vi "Format Display to Uncertainty.vi"(5 "- uncertainty reference":refnum<vi>, 7 "+ uncertainty reference":refnum<vi>, 8 "error in (no error)":errorcluster, 11 "value reference":refnum<vi>) -> (0 "error out":errorcluster, 3 "formatting string":string)   [LabVIEW 2013, in "varilib.lvlib"]
doc: "Sets format of referenced numeric control according the positive or both positive or negative uncertainties of referenced numeric controls. Format is done to the order of two significant numbers of smaller uncertainty. A formatting string is returned in the output."
uses:
  varilib.lvlib
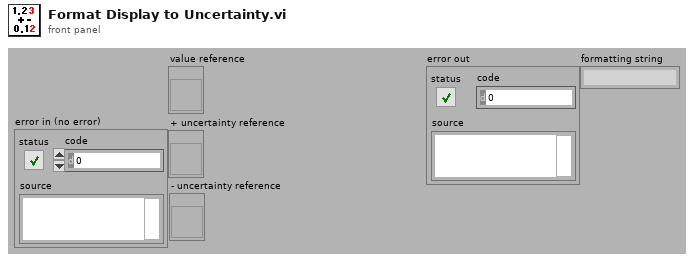
[diagram p1: front panel]
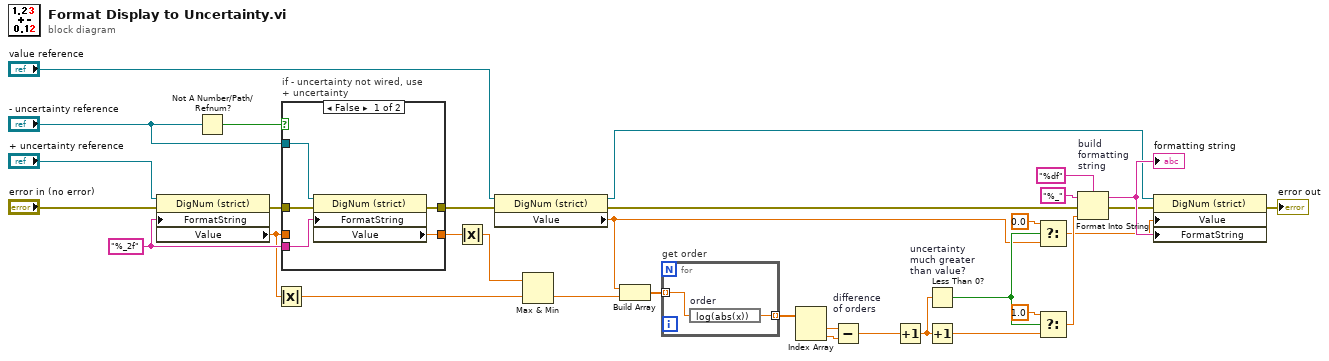
[diagram p0: block diagram]
diagram:
  w16 = "%_2f" ("Format String")
  n1 = property class="DigNum (strict)"(reference="+ uncertainty reference", error in="error in (no error)", "FormatString"=w16) -> (error out=w9:errorcluster, "Value"=w2:dbl)  [unwired: 1 out]
  n2 = Not A Number/Path/Refnum?(number/path/refnum="- uncertainty reference") -> (NaN/Path/Refnum?=w3:bool)
  n3 = Absolute Value(x=w2) -> (abs(x)=w14:dbl)
  n4 = case "if - uncertainty not wired, use \n+ uncertainty" shown="False" w3 {
    tunnel: w16 -> [w38 _]
    tunnel: [w37 w39] -> w15
    tunnel: w9 -> [w36 w40]
    tunnel: [w35 w40] -> w8
    tunnel: w2 -> [_ w39]
    tunnel: "- uncertainty reference" -> [w34 _]
    frame False {
      n5 = property class="DigNum (strict)"(reference=w34, error in=w36, "FormatString"=w38) -> (error out=w35:errorcluster, "Value"=w37:dbl)  [unwired: 1 out]
    }
    frame True {
    }
  }
  n6 = Absolute Value(x=w15) -> (abs(x)=w30:dbl)
  n7 = property class="DigNum (strict)"(reference="value reference", error in=w8) -> (reference out=w11:refnum<vi>, error out=w7:errorcluster, "Value"=w12:dbl)
  n8 = Max & Min(x=w30, y=w14) -> (min(x,y)=w13:dbl)  [unwired: 1 out]
  n9 = Build Array(w12, w13) -> (w27:dbl[])
  n10 = for "get order" {
    tunnel: [w41] -> w26 mode=indexing
    tunnel: w27 -> [w42] mode=indexing
    n11 = expression code="log(abs(x))" "order"(w42) -> (w41:dbl)
  }
  n12 = Index Array(array=w26) -> (element #1=w25:dbl, element #2=w24:dbl)  [unwired: 2 in]
  n13 = Subtract "difference\nof orders"(x=w25, y=w24) -> (x-y=w23:dbl)
  n14 = Increment(x=w23) -> (x+1=w17:dbl)
  n15 = Less Than 0? "uncertainty\nmuch greater\nthan value?"(x=w17) -> (x < 0?=w20:bool)
  n16 = Increment(x=w17) -> (x+1=w19:dbl)
  n17 = Select(t=0.0, s=w20, f=w12) -> (s? t:f=w10:dbl)
  n18 = Select(t=1.0, s=w20, f=w19) -> (s? t:f=w21:dbl)
  n19 = Format Into String "build\nformatting\nstring"(format string="%df", initial string="%_", error in=w7, w21) -> (resulting string=w31:string, error out=w6:errorcluster)
  "formatting string" <- w31
  n20 = property class="DigNum (strict)"(reference=w11, error in=w6, "Value"=w10, "FormatString"=w31) -> (error out=→"error out":errorcluster)  [unwired: 1 out]
